vi "Configure AMQP Client.vi"(8 "error in (no error)":errorcluster, 11 "Logger in":refnum<class "Logger.lvclass">) -> (0 "error out":errorcluster, 3 "Logger out":refnum<class "Logger.lvclass">)   [LabVIEW 2026, in "Logger.lvlib" / "Logger.lvclass"]
uses:
  Logger.lvclass
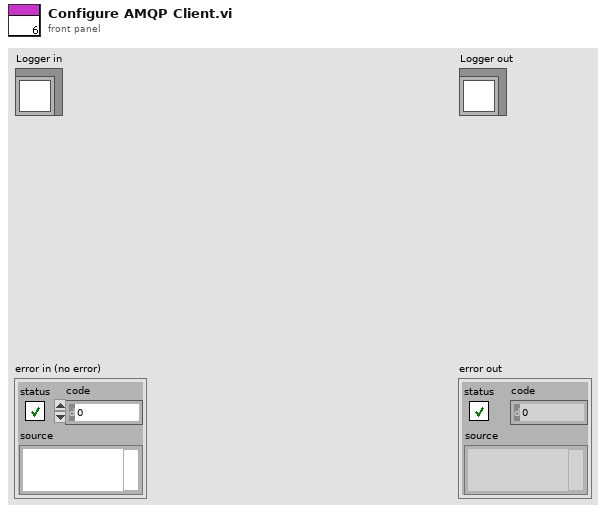
[diagram p1: front panel]
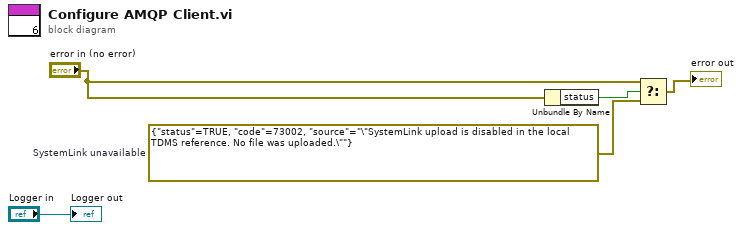
[diagram p0: block diagram]
diagram:
  w3 = errorcluster {"status"=TRUE, "code"=73002, "source"="\"SystemLink upload is disabled in the local TDMS reference. No file was uploaded.\""}  # SystemLink unavailable
  n1 = Unbundle By Name("error in (no error)") -> ("status"=w5:bool)
  n2 = Select(t="error in (no error)", s=w5, f=w3) -> (s? t:f=→"error out":errorcluster)
  "Logger out" <- "Logger in"
